vi "RGseriesSeria19531Ceramic.vi"() -> ()   [LabVIEW 2015]
uses:
  <vilib>/Instr/_visa.llb/VISA Configure Serial Port (Instr).vi
  <userlib>/caLab/Private/Get_PV-1D.vi
  <userlib>/caLab/Private/Get_PV.vi
  <userlib>/caLab/Private/Put_DBL-1D_PV-1D.vi
panel:
  in  "Ifactor":dbl=33.3
  in  "APX:PS2_T_RV":dbl
  out "APX:PS2_V_EV":dbl format="%.3f"
  out "APX:PS2_I_EV":dbl format="%.3f"
  out "Ilim_factor":dbl
  out "Vlim_factor":dbl
  out "SSE:Tsample":dbl
  in  "I lower limit":dbl
  in  "V lower limit":dbl
  in  "I upper limit":dbl=2.8
  in  "V upper limit":dbl=18.0
  out "APX:PS2_Ct":dbl
  out "APX:PS2_Rzero":dbl
  in  "Heater":u16(ring) items=["Ceramic W/Mo", "Kanthal A-1"]
  out "APX:Theater":dbl
  out "APX:PS2_R_MV":dbl format="%.2f"
  out "PS1:R_MV":dbl format="%.2f"
  out "APX:Tpiezo":dbl
  in  "REMOTE/LOCAL":bool
  out "APX:Tcopper":dbl
  in  "Timer1":bool
  in  "Reset Timer1":bool=TRUE caption="Auto Reset"
  out "Time has Elapsed":bool
  in  "Time Target1 (min)":dbl=1.0 caption="Time Target (s)"
  out "Elapsed Time (min)":dbl caption="Elapsed Time (s)"
  in  "PS1:I_RV":dbl min=0.0 max=0.5 step=0.01
  in  "PS1:V_RV":dbl min=0.0 max=5.0 step=0.01
  out "PS1:P_MV":dbl format="%.2f"
  out "PS1:I_MV":dbl format="%.3g"
  out "PS1:V_MV":dbl format="%.3g"
  in  "PS1:OUT":bool
  out "APX:Thpc OK?":bool
  out "APX:Tpiezo OK?":bool
  out "PS2_P_MV":dbl format="%.2f"
  in  "APX:PS2_I_RV":dbl min=0.0 max=0.5 step=0.002
  in  "APX:PS2_OUT":bool
  in  "stop":bool
  out "APX:PS2_I_MV":dbl format="%.3g"
  out "APX:PS2_V_MV":dbl format="%.3g"
  in  "VISA resource name":refnum<visa-resource-name>="COM12"
  in  "APX:PS2_V_RV":dbl min=0.0 max=8.0 step=0.05
  # "Sample Heater Control"
  # "Copper mesh temperature control"
  # "COM12"
  # "V"
  # "V"
  # "A"
  # "A"
  # "Max 1.2A/0.4x0.1wire"
  # "W"
  # "ohm"
  # "W"
  # "ohm"
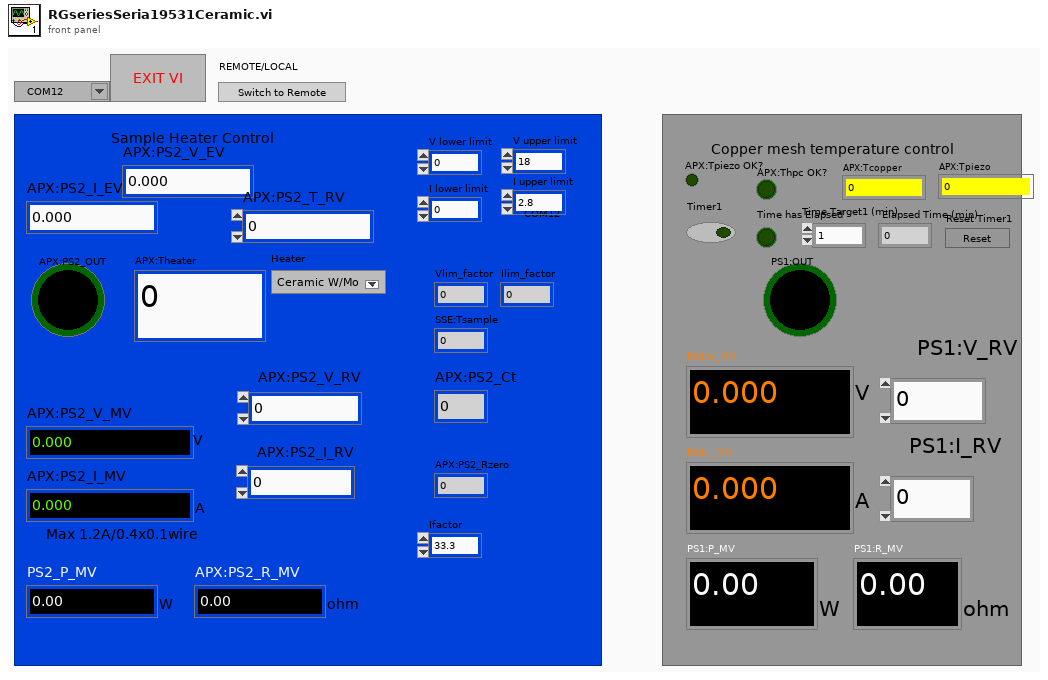
[diagram p1: front panel]
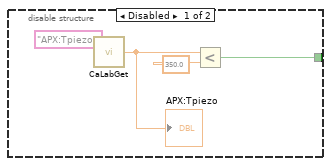
[diagram p2: hidden frame]
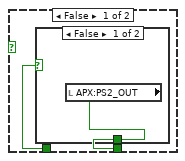
[diagram p4: hidden frame]
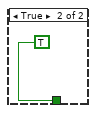
[diagram p5: hidden frame]
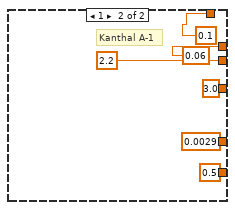
[diagram p6: hidden frame]
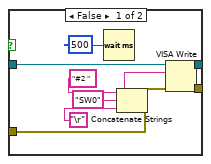
[diagram p7: hidden frame]
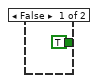
[diagram p9: hidden frame]
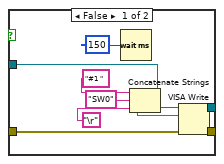
[diagram p10: hidden frame]
diagram:
  w46 = u16 0 items=["None", "XON/XOFF", "RTS/CTS", "XON/XOFF & RTS/CTS", "DTR/DSR", "XON/XOFF & DTR/DSR"] ("flow control (0:none)")
  w47 = u16 10 items=["1.0"=10, "1.5"=15, "2.0"=20] ("stop bits (10: 1 bit)")
  # "enable output"
  # "disable remote control"
  # "OpenComport"
  # "Stop bits"
  # "enable remote control"
  # "enable output"
  n1 = Concatenate Strings("#2 " ("initial string"), "REN" ("string"), "\r") -> (w45:string)
  n2 = call-poly "VISA Configure Serial Port"("VISA resource name"=refnum<visa-resource-name> "COM20", "timeout (10sec)"=u32 10000, "baud rate (9600)"=u32 9600, "data bits (8)"=u16 8, "parity (0:none)"=enum16{"None", "Odd", "Even", "Mark", "Space"}."None", "stop bits (10: 1 bit)"=w47, "flow control (0:none)"=w46) -> ("VISA resource name out"=w42:refnum<visa-resource-name>, "error out"=w41:errorcluster)  [unwired: 7 in]
  n3 = VISA Write(VISA resource name=w42, write buffer=w45, error in (no error)=w41) -> (VISA resource name out=w11:refnum<visa-resource-name>, error out=w4:errorcluster)  [unwired: 1 out]
  n4 = flat-sequence {
    tunnel: w4 -> [w60]
    tunnel: [w60] -> w5
    frame #0 {
      n5 = Wait (ms)(milliseconds to wait=u32 500) -> ()  [unwired: 1 out]
    }
  }
  n6 = Concatenate Strings("#1 " ("initial string"), "REN" ("string"), "\r") -> (w6:string)
  n7 = VISA Write(VISA resource name=w11, write buffer=w6, error in (no error)=w5) -> (VISA resource name out=w10:refnum<visa-resource-name>, error out=w3:errorcluster)  [unwired: 1 out]
  n8 = flat-sequence {
    tunnel: [w64] -> w28
    tunnel: w3 -> [w64]
    frame #0 {
      n9 = Wait (ms)(milliseconds to wait=u32 500) -> ()  [unwired: 1 out]
      n10 = property on="APX:PS2_V_RV" class="DigNum (strict)"("Value"=0.0 ("VCN_REQ")) -> ()  [unwired: 2 in, 2 out]
      n11 = property on="APX:PS2_I_RV" class="DigNum (strict)"("Value"=0.0 ("APX:RG183_I_RV")) -> ()  [unwired: 2 in, 2 out]
    }
  }
  n12 = local write "REMOTE/LOCAL"(FALSE ("REMOTE/LOCAL")) -> ()
  n13 = Concatenate Strings("#2 " ("format string"), "SW0" ("initial string"), "\r" ("input 1")) -> (w44:string)
  n14 = VISA Write(VISA resource name=w10, write buffer=w44, error in (no error)=w28) -> (VISA resource name out=w30:refnum<visa-resource-name>, error out=w29:errorcluster)  [unwired: 1 out]
  n15 = while {
    tunnel: w30 -> [w74]
    tunnel: w29 -> [w75]
    tunnel: [w71] -> w27
    tunnel: [w70] -> w26
    stop <- "stop" stop-if-true
    n16 = flat-sequence {
      tunnel: w74 -> [w85]
      tunnel: w75 -> [w86]
      tunnel: [w86] -> w68
      tunnel: [w85] -> w67
      tunnel: [w167] -> w73
      tunnel: [w166] -> w72
      tunnel: w68 -> [w165]
      tunnel: w67 -> [w163]
      tunnel: w73 -> [w301]
      tunnel: w72 -> [w298]
      tunnel: [w279] -> w66
      tunnel: [w278] -> w65
      tunnel: [w395] -> w70
      tunnel: [w396] -> w71
      tunnel: w66 -> [w396]
      tunnel: w65 -> [w395]
      frame #0 {
        n17 = disable-structure shown="Enabled" {
          disable-tunnel: [w87 TRUE ("APX:Tpiezo OK?")] -> w78
          frame Disabled {
            n18 = call-poly "CaLabGet.vi"("PV Name"="APX:Tpiezo") -> ("1rst Value (number)"=w89:dbl)  [unwired: 8 in, 6 out]
            "APX:Tpiezo" <- w89
            n19 = Less?(x=w89, y=350.0) -> (x < y?=w87:bool)
          }
          frame Enabled {
          }
        }
        "APX:Tpiezo OK?" <- w78
        n20 = case shown="0, Default" "Heater" {
          tunnel: [0.00483 ("APX:PS2_Ct") 0.0029 ("APX:PS2_Ct")] -> w81
          tunnel: [9.3 ("APX:PS2_Rzero") 0.5 ("APX:PS2_Rzero")] -> w82
          tunnel: [0.5 2.2] -> w83
          tunnel: [10.0 3.0] -> w84
          tunnel: [0.1 0.1] -> w77
          tunnel: [0.06 0.06] -> w76
          frame 0, Default {
            (unwired) 9.89 ("APX:PS2_Rzero")
            (unwired) 0.0325 ("APX:PS2_Ct")
            (unwired) 6.21 ("APX:PS2_Rzero")
            # "W/Mo"
          }
          frame 1 {
            # "Kanthal A-1"
          }
        }
        n21 = case shown="True" "REMOTE/LOCAL" {
          frame False {
          }
          frame True {
            w94 = 0 ("disabled index (col)")
            (unwired) "APX:Thpc"
            n22 = call-poly "CaLabGet.vi"("PV Names"=string[] ["APX:PS2_V_RV", "APX:PS2_I_RV", "APX:PS2_OUT_1", "APX:PS2_OUT_0", "SSE:Tsample"]) -> ("Value Array (number)"=w93:dbl[][])  [unwired: 8 in, 6 out]
            n23 = Index Array(array=w93, index (row)=4, index (col)=w94) -> (element=→"SSE:Tsample":dbl)
            n24 = Index Array(array=w93, index (row)=2, index (col)=w94) -> (element=w107:dbl)
            n25 = Index Array(array=w93, index (row)=0, index (col)=w94) -> (element=w97:dbl)
            n26 = Index Array(array=w93, index (row)=1, index (col)=w94) -> (element=w96:dbl)
            n27 = Index Array(array=w93, index (row)=3 ("disabled index (row)"), index (col)=w94) -> (element=w101:dbl)
            n28 = Number To Boolean Array(number=w107) -> (Boolean array=w106:bool[])
            n29 = Number To Boolean Array(number=w101) -> (Boolean array=w103:bool[])
            n30 = local write "APX:PS2_I_RV"(w96) -> ()
            n31 = Index Array(array=w106, index=0) -> (element=w99:bool)
            n32 = local write "APX:PS2_V_RV"(w97) -> ()
            n33 = Index Array(array=w103, index=0) -> (element=w100:bool)
            n34 = case shown="True" w100 {
              tunnel: w99 -> [w113 _]
              tunnel: [w112 FALSE] -> w98
              frame False {
                n35 = case shown="False" w113 {
                  tunnel: [w114 TRUE] -> w112
                  frame False {
                    n36 = local read "APX:PS2_OUT"() -> (w114:bool)
                  }
                  frame True {
                  }
                }
              }
              frame True {
              }
            }
            n37 = local write "APX:PS2_OUT"(w98) -> ()
          }
        }
        n38 = local write "I upper limit"(w83) -> ()
        n39 = local write "V upper limit"(w84) -> ()
        n40 = local write "APX:PS2_Ct"(w81) -> ()
        n41 = local write "APX:PS2_Rzero"(w82) -> ()
        n42 = local write "V lower limit"(w77) -> ()
        n43 = local write "I lower limit"(w76) -> ()
      }
      frame #1 {
        w139 = 293.0 ("y")
        # "measure current"
        # "measure voltage"
        # "measure voltage"
        # "measure curent"
        # "Measured Voltage"
        # "Measured Current"
        # "Set current"
        # "Set voltage"
        # "disable output"
        n44 = local read "APX:PS2_Rzero"() -> (w134:dbl)
        n45 = local read "APX:PS2_R_MV"() -> (w152:dbl)
        n46 = In Range and Coerce(upper limit=65.0, x=w152, lower limit=w134) -> (coerced(x)=w150:dbl)  [unwired: 1 out]
        n47 = Divide(x=w150, y=w134) -> (x/y=w149:dbl)
        n48 = Subtract(x="APX:PS2_T_RV", y=w139) -> (x-y=w133:dbl)
        n49 = Subtract(x=w149, y=1.0) -> (x-y=w147:dbl)
        n50 = local read "APX:PS2_Ct"() -> (w138:dbl)
        n51 = Multiply(x=w133, y=w138) -> (x*y=w137:dbl)
        n52 = Divide(x=w147, y=w138) -> (x/y=w146:dbl)
        n53 = Add(x=w137, y=1.0) -> (x+y=w135:dbl)
        n54 = Multiply(x=w135, y=w134) -> (x*y=w130:dbl)
        n55 = Multiply(x=w133, y=0.02) -> (x*y=w129:dbl)
        "APX:PS2_V_EV" <- w129
        n56 = Add(x=w146, y=w139) -> (x+y=→"APX:Theater":dbl)
        n57 = Divide(x=w129, y=w130) -> (x/y=→"APX:PS2_I_EV":dbl)
        n58 = case shown="True" "APX:PS2_OUT" {
          tunnel: w163 -> [w233 w242]
          tunnel: w165 -> [w232 w241]
          tunnel: [w231 w240] -> w164
          tunnel: [w230 w239] -> w162
          frame False {
            n59 = Wait (ms)(milliseconds to wait=u32 500) -> ()  [unwired: 1 out]
            n60 = Concatenate Strings("#2 " ("format string"), "SW0" ("initial string"), "\r" ("input 1")) -> (w235:string)
            n61 = VISA Write(VISA resource name=w233, write buffer=w235, error in (no error)=w232) -> (VISA resource name out=w230:refnum<visa-resource-name>, error out=w231:errorcluster)  [unwired: 1 out]
          }
          frame True {
            n62 = Wait (ms)(milliseconds to wait=u32 500) -> ()  [unwired: 1 out]
            n63 = Concatenate Strings("#2 " ("format string"), "SW1" ("initial string"), "\r" ("input 1")) -> (w244:string)
            n64 = VISA Write(VISA resource name=w242, write buffer=w244, error in (no error)=w241) -> (VISA resource name out=w239:refnum<visa-resource-name>, error out=w240:errorcluster)  [unwired: 1 out]
          }
        }
        n65 = In Range and Coerce(upper limit="V upper limit", x="APX:PS2_V_RV", lower limit="V lower limit") -> (coerced(x)=w160:dbl)  [unwired: 1 out]
        n66 = flat-sequence {
          tunnel: w162 -> [w260]
          tunnel: w164 -> [w261]
          tunnel: [w261] -> w168
          tunnel: [w260] -> w169
          frame #0 {
            n67 = Wait (ms)(milliseconds to wait=u32 500) -> ()  [unwired: 1 out]
          }
        }
        n68 = Multiply(x=5.5, y=w160) -> (x*y=w227:dbl)
        n69 = Number To Fractional String(number=w227, width (-)=i16 5, precision (6)=i16 2) -> (F-format string=w228:string)  [unwired: 1 in]
        n70 = Concatenate Strings("#2" ("format string"), "VCN " ("initial string"), w228, "\r") -> (w173:string)
        n71 = Concatenate Strings("#2 " ("format string"), "VM" ("initial string"), "\r" ("input 1")) -> (w204:string)
        n72 = VISA Write(VISA resource name=w169, write buffer=w173, error in (no error)=w168) -> (VISA resource name out=w203:refnum<visa-resource-name>, error out=w202:errorcluster)  [unwired: 1 out]
        n73 = VISA Write(VISA resource name=w203, write buffer=w204, error in (no error)=w202) -> (VISA resource name out=w189:refnum<visa-resource-name>, error out=w187:errorcluster)  [unwired: 1 out]
        n74 = flat-sequence {
          tunnel: w189 -> [w259]
          tunnel: [w259] -> w188
          tunnel: w187 -> [w258]
          tunnel: [w258] -> w186
          frame #0 {
            n75 = Wait (ms)(milliseconds to wait=u32 500) -> ()  [unwired: 1 out]
          }
        }
        n76 = In Range and Coerce(upper limit="I upper limit", x="APX:PS2_I_RV", lower limit="I lower limit") -> (coerced(x)=w158:dbl)  [unwired: 1 out]
        n77 = property class="Instr"(reference=w188, error in=w186) -> (reference out=w195:refnum<visa-resource-name>, error out=w194:errorcluster, "Serial Settings:Number of Bytes at Serial Port"=w193:u32)
        n78 = Multiply(x=33.0, y=w158) -> (x*y=w217:dbl)
        n79 = Number To Fractional String(number=w217, width (-)=i16 5, precision (6)=i16 2) -> (F-format string=w220:string)  [unwired: 1 in]
        n80 = VISA Read(VISA resource name=w195, byte count=w193, error in (no error)=w194) -> (VISA resource name out=w181:refnum<visa-resource-name>, read buffer=w174:string, error out=w180:errorcluster)  [unwired: 1 out]
        n81 = Concatenate Strings("#2 " ("initial string"), "ICN " ("initial string"), w220, "\r") -> (w172:string)
        n82 = flat-sequence {
          tunnel: w181 -> [w252]
          tunnel: w180 -> [w251]
          tunnel: [w252] -> w178
          tunnel: [w251] -> w179
          frame #0 {
            n83 = Wait (ms)(milliseconds to wait=u32 500) -> ()  [unwired: 1 out]
          }
        }
        n84 = String Subset(string=w174, offset (0)=3) -> (substring=w171:string)  [unwired: 1 in]
        n85 = Concatenate Strings("#2 " ("format string"), "IM" ("initial string"), "\r" ("input 1")) -> (w197:string)
        n86 = VISA Write(VISA resource name=w178, write buffer=w172, error in (no error)=w179) -> (VISA resource name out=w199:refnum<visa-resource-name>, error out=w200:errorcluster)  [unwired: 1 out]
        n87 = Fract/Exp String To Number(string=w171) -> (number=w213:dbl)  [unwired: 3 in, 1 out]
        n88 = VISA Write(VISA resource name=w199, write buffer=w197, error in (no error)=w200) -> (VISA resource name out=w185:refnum<visa-resource-name>, error out=w184:errorcluster)  [unwired: 1 out]
        n89 = Divide(x=w213, y=5.5 ("x")) -> (x/y=w155:dbl)
        "APX:PS2_V_MV" <- w155
        n90 = flat-sequence {
          tunnel: w185 -> [w255]
          tunnel: w184 -> [w254]
          tunnel: [w255] -> w183
          tunnel: [w254] -> w182
          frame #0 {
            n91 = Wait (ms)(milliseconds to wait=u32 500) -> ()  [unwired: 1 out]
          }
        }
        n92 = property class="Instr"(reference=w183, error in=w182) -> (reference out=w192:refnum<visa-resource-name>, error out=w191:errorcluster, "Serial Settings:Number of Bytes at Serial Port"=w190:u32)
        n93 = VISA Read(VISA resource name=w192, byte count=w190, error in (no error)=w191) -> (VISA resource name out=w177:refnum<visa-resource-name>, read buffer=w175:string, error out=w176:errorcluster)  [unwired: 1 out]
        n94 = flat-sequence {
          tunnel: w177 -> [w249]
          tunnel: w176 -> [w248]
          tunnel: [w249] -> w167
          tunnel: [w248] -> w166
          frame #0 {
            n95 = Wait (ms)(milliseconds to wait=u32 500) -> ()  [unwired: 1 out]
          }
        }
        n96 = String Subset(string=w175, offset (0)=3) -> (substring=w170:string)  [unwired: 1 in]
        n97 = Fract/Exp String To Number(string=w170) -> (number=w210:dbl)  [unwired: 3 in, 1 out]
        n98 = Divide(x=w210, y=33.5 ("x")) -> (x/y=w156:dbl)
        "APX:PS2_I_MV" <- w156
        n99 = Multiply(x=w155, y=w156) -> (x*y=→"PS2_P_MV":dbl)
        n100 = Divide(x=w155, y=w156) -> (x/y=→"APX:PS2_R_MV":dbl)
      }
      frame #2 {
        (unwired) 33.3 ("x")
        (unwired) 37.35 ("x")
        # "measure curent"
        # "Measured Voltage"
        # "Measured Current"
        # "disable output"
        # "measure current"
        # "measure voltage"
        # "Set current"
        # "measure voltage"
        # "Set voltage"
        n101 = case shown="True" "Reset Timer1" {
          frame False {
          }
          frame True {
            n102 = property on="Elapsed Time (min)" class="DigNum (strict)"("Value"=0.0 ("Elapsed Time (min)")) -> ()  [unwired: 2 in, 2 out]
          }
        }
        n103 = case shown="True" "Timer1" {
          tunnel: "Time Target1 (min)" -> [_ w356]
          tunnel: [TRUE w355] -> w269
          frame False {
          }
          frame True {
            w360 = 60.0 ("y")
            n104 = Multiply(x=w356, y=w360) -> (x*y=w358:dbl)
            n105 = call "Elapsed Time"("Time Target (s)"=w358) -> ("Elapsed Time (s)"=w359:dbl, "Time has Elapsed"=w357:bool)  [unwired: 11 in, 6 out]
            "Time has Elapsed" <- w357
            n106 = Divide(x=w359, y=w360) -> (x/y=→"Elapsed Time (min)":dbl)
            n107 = Not(x=w357) -> (.not. x?=w355:bool)
          }
        }
        n108 = call-poly "CaLabGet.vi"("PV Name"="APX:Tcopper") -> ("1rst Value (number)"=w351:dbl)  [unwired: 8 in, 6 out]
        "APX:Tcopper" <- w351
        n109 = Less?(x=w351, y=420.0) -> (x < y?=w300:bool)
        "APX:Thpc OK?" <- w300
        n110 = And(x=w300, y="PS1:OUT") -> (x .and. y?=w273:bool)
        n111 = And(x=w273, y=w269) -> (x .and. y?=w272:bool)
        n112 = case shown="True" w272 {
          tunnel: w301 -> [w374 w383]
          tunnel: w298 -> [w373 w382]
          tunnel: [w372 w381] -> w297
          tunnel: [w371 w380] -> w296
          frame False {
            n113 = Wait (ms)(milliseconds to wait=u32 150) -> ()  [unwired: 1 out]
            n114 = Concatenate Strings("#1 " ("format string"), "SW0" ("initial string"), "\r" ("input 1")) -> (w378:string)
            n115 = VISA Write(VISA resource name=w374, write buffer=w378, error in (no error)=w373) -> (VISA resource name out=w371:refnum<visa-resource-name>, error out=w372:errorcluster)  [unwired: 1 out]
          }
          frame True {
            n116 = Wait (ms)(milliseconds to wait=u32 500) -> ()  [unwired: 1 out]
            n117 = Concatenate Strings("#1 " ("format string"), "SW1" ("initial string"), "\r" ("input 1")) -> (w387:string)
            n118 = VISA Write(VISA resource name=w383, write buffer=w387, error in (no error)=w382) -> (VISA resource name out=w380:refnum<visa-resource-name>, error out=w381:errorcluster)  [unwired: 1 out]
          }
        }
        n119 = In Range and Coerce(upper limit=5.01, x="PS1:V_RV", lower limit=0.0) -> (coerced(x)=w313:dbl)  [unwired: 1 out]
        n120 = flat-sequence {
          tunnel: [w390] -> w294
          tunnel: w297 -> [w390]
          tunnel: [w389] -> w295
          tunnel: w296 -> [w389]
          frame #0 {
            n121 = Wait (ms)(milliseconds to wait=u32 500) -> ()  [unwired: 1 out]
          }
        }
        n122 = Multiply(x=5.55, y=w313) -> (x*y=w304:dbl)
        n123 = Number To Fractional String(number=w304, width (-)=i16 5, precision (6)=i16 2) -> (F-format string=w303:string)  [unwired: 1 in]
        n124 = Concatenate Strings("#1" ("format string"), "VCN " ("initial string"), w303, "\r") -> (w318:string)
        n125 = Concatenate Strings("#1" ("format string"), "VM" ("initial string"), "\r" ("input 1")) -> (w317:string)
        n126 = VISA Write(VISA resource name=w295, write buffer=w318, error in (no error)=w294) -> (VISA resource name out=w319:refnum<visa-resource-name>, error out=w345:errorcluster)  [unwired: 1 out]
        n127 = VISA Write(VISA resource name=w319, write buffer=w317, error in (no error)=w345) -> (VISA resource name out=w346:refnum<visa-resource-name>, error out=w347:errorcluster)  [unwired: 1 out]
        n128 = flat-sequence {
          tunnel: w346 -> [w394]
          tunnel: [w394] -> w348
          tunnel: w347 -> [w393]
          tunnel: [w393] -> w349
          frame #0 {
            n129 = Wait (ms)(milliseconds to wait=u32 500) -> ()  [unwired: 1 out]
          }
        }
        n130 = property class="Instr"(reference=w348, error in=w349) -> (reference out=w341:refnum<visa-resource-name>, error out=w342:errorcluster, "Serial Settings:Number of Bytes at Serial Port"=w343:u32)
        n131 = VISA Read(VISA resource name=w341, byte count=w343, error in (no error)=w342) -> (VISA resource name out=w277:refnum<visa-resource-name>, read buffer=w344:string, error out=w275:errorcluster)  [unwired: 1 out]
        n132 = flat-sequence {
          tunnel: w277 -> [w364]
          tunnel: [w364] -> w276
          tunnel: [w362] -> w274
          tunnel: w275 -> [w362]
          frame #0 {
            n133 = Wait (ms)(milliseconds to wait=u32 500) -> ()  [unwired: 1 out]
          }
        }
        n134 = String Subset(string=w344, offset (0)=3) -> (substring=w333:string)  [unwired: 1 in]
        n135 = In Range and Coerce(upper limit=0.501, x="PS1:I_RV", lower limit=0.0) -> (coerced(x)=w337:dbl)  [unwired: 1 out]
        n136 = Fract/Exp String To Number(string=w333) -> (number=w327:dbl)  [unwired: 3 in, 1 out]
        n137 = Multiply(x="Ifactor", y=w337) -> (x*y=w323:dbl)
        n138 = Number To Fractional String(number=w323, width (-)=i16 5, precision (6)=i16 2) -> (F-format string=w321:string)  [unwired: 1 in]
        n139 = Concatenate Strings("#1 " ("initial string"), "ICN " ("initial string"), w321, "\r") -> (w338:string)
        n140 = Concatenate Strings("#1 " ("format string"), "IM" ("initial string"), "\r" ("input 1")) -> (w339:string)
        n141 = VISA Write(VISA resource name=w276, write buffer=w338, error in (no error)=w274) -> (VISA resource name out=w340:refnum<visa-resource-name>, error out=w263:errorcluster)  [unwired: 1 out]
        n142 = flat-sequence {
          tunnel: w282 -> [w369]
          tunnel: w281 -> [w368]
          tunnel: [w369] -> w288
          tunnel: [w368] -> w287
          frame #0 {
            n143 = Wait (ms)(milliseconds to wait=u32 500) -> ()  [unwired: 1 out]
          }
        }
        n144 = VISA Write(VISA resource name=w340, write buffer=w339, error in (no error)=w263) -> (VISA resource name out=w282:refnum<visa-resource-name>, error out=w281:errorcluster)  [unwired: 1 out]
        n145 = property class="Instr"(reference=w288, error in=w287) -> (reference out=w291:refnum<visa-resource-name>, error out=w290:errorcluster, "Serial Settings:Number of Bytes at Serial Port"=w289:u32)
        n146 = VISA Read(VISA resource name=w291, byte count=w289, error in (no error)=w290) -> (VISA resource name out=w286:refnum<visa-resource-name>, read buffer=w284:string, error out=w285:errorcluster)  [unwired: 1 out]
        n147 = flat-sequence {
          tunnel: w286 -> [w366]
          tunnel: w285 -> [w365]
          tunnel: [w366] -> w279
          tunnel: [w365] -> w278
          frame #0 {
            n148 = Wait (ms)(milliseconds to wait=u32 500) -> ()  [unwired: 1 out]
          }
        }
        n149 = String Subset(string=w284, offset (0)=3) -> (substring=w283:string)  [unwired: 1 in]
        n150 = Fract/Exp String To Number(string=w283) -> (number=w293:dbl)  [unwired: 3 in, 1 out]
        n151 = Divide(x=w327, y=5.55 ("x")) -> (x/y=w267:dbl)
        "PS1:V_MV" <- w267
        n152 = Divide(x=w293, y="Ifactor") -> (x/y=w266:dbl)
        "PS1:I_MV" <- w266
        n153 = Divide(x=w267, y=w266) -> (x/y=→"PS1:R_MV":dbl)
        n154 = Multiply(x=w267, y=w266) -> (x*y=→"PS1:P_MV":dbl)
      }
      frame #3 {
        n155 = flat-sequence {
          frame #0 {
            w401 = 0.0 ("element")
            n156 = local read "APX:PS2_OUT"() -> (w405:bool)
            n157 = local read "APX:PS2_R_MV"() -> (w410:dbl)
            n158 = local read "APX:PS2_V_MV"() -> (w408:dbl)
            n159 = local read "APX:PS2_I_MV"() -> (w409:dbl)
            n160 = local read "APX:Theater"() -> (w411:dbl)
            n161 = Boolean To (0,1)(Boolean=w405) -> (0, 1=w404:i16)
            n162 = local read "APX:PS2_Rzero"() -> (w397:dbl)
            n163 = Build Array("APX:Theater", "APX:PS2_R_MV", "APX:PS2_I_MV", "APX:PS2_V_MV", "APX:PS2_OUT", "APX:PS2_OUT_0", "APX:PS2_OUT_1", "APX:PS2_Rzero", "APX:PS2_Ct") -> (w416:string[])
            n164 = local read "APX:PS2_Ct"() -> (w398:dbl)
            n165 = Build Array(w411, w410, w409, w408, w404, w401, w401, w397, w398) -> (w407:dbl[])
            n166 = call-poly <userlib>:"CaLabPut.vi"("Values"=w407, "PV Names"=w416) -> ()  [unwired: 6 in, 4 out]
          }
        }
      }
    }
  }
  n167 = Concatenate Strings("#2 " ("format string"), "SW0" ("initial string"), "\r" ("input 1")) -> (w36:string)
  n168 = VISA Write(VISA resource name=w27, write buffer=w36, error in (no error)=w26) -> (VISA resource name out=w32:refnum<visa-resource-name>, error out=w31:errorcluster)  [unwired: 1 out]
  n169 = Concatenate Strings("#2 " ("initial string"), "\r", "GTL" ("input 1")) -> (w43:string)
  n170 = VISA Write(VISA resource name=w32, write buffer=w43, error in (no error)=w31) -> (VISA resource name out=w15:refnum<visa-resource-name>, error out=w14:errorcluster)  [unwired: 1 out]
  n171 = Concatenate Strings("#1 " ("format string"), "SW0" ("initial string"), "\r" ("input 1")) -> (w21:string)
  n172 = VISA Write(VISA resource name=w15, write buffer=w21, error in (no error)=w14) -> (VISA resource name out=w17:refnum<visa-resource-name>, error out=w16:errorcluster)  [unwired: 1 out]
  n173 = Concatenate Strings("#1" ("initial string"), "\r", "GTL" ("input 1")) -> (w22:string)
  n174 = VISA Write(VISA resource name=w17, write buffer=w22, error in (no error)=w16) -> (VISA resource name out=w13:refnum<visa-resource-name>, error out=w12:errorcluster)  [unwired: 1 out]
  n175 = flat-sequence {
    tunnel: w13 -> [w421]
    tunnel: w12 -> [w420]
    tunnel: [w421] -> w38
    tunnel: [w420] -> w37
    frame #0 {
      n176 = Wait (ms)(milliseconds to wait=u32 500) -> ()  [unwired: 1 out]
      n177 = property on="APX:PS2_OUT" class="Bool (strict)"("Value"=FALSE ("Output")) -> ()  [unwired: 2 in, 2 out]
      n178 = property on="APX:PS2_V_RV" class="DigNum (strict)"("Value"=0.0 ("VCN_REQ")) -> ()  [unwired: 2 in, 2 out]
      n179 = property on="APX:PS2_I_RV" class="DigNum (strict)"("Value"=0.0 ("APX:RG183_I_RV")) -> ()  [unwired: 2 in, 2 out]
    }
  }
  n180 = VISA Close(VISA resource name=w38, error in (no error)=w37) -> ()  [unwired: 1 out]
